vi "RT Driver VI.vi"(6 "Device Clock":string, 9 "Device Inputs FIFO":refnum<k33>, 10 "Device Outputs FIFO":refnum<k33>, 11 "Device Reference":T1 format="%.0x") -> ()   [LabVIEW 2019, in "DeltaPSControl Engine.lvlib"]
uses:
  DeltaPSControl Engine.lvlib
  <vilib>/NI VeriStand/Custom Device API/Custom Device Item Ref.ctl
  <vilib>/NI VeriStand/Custom Device API/Custom Device Channel Type.ctl
  <vilib>/NI VeriStand/Custom Device API/Message Response (String).ctl
  <vilib>/NI VeriStand/Custom Device API/Message Response (Byte Array).ctl
  Shared/Constants.vi
  <vilib>/NI VeriStand/Custom Device API/Get Item Property (String Array).vi
  <vilib>/NI VeriStand/Custom Device API/Get Item Property (String).vi
  <vilib>/NI VeriStand/Custom Device API/Get Item Property (U16).vi
  <vilib>/NI VeriStand/Custom Device API/Custom Device API.lvlib
  <vilib>/NI VeriStand/Custom Device Tools/Custom Device Utility Library/Custom Device Utility Library.lvlib
  Shared/DeltaPSControl Shared.lvlib
panel:
  out "idn/pud":string
  in  "Initialization Status Notifier":refnum<notifier>
  in  "Status Notifier":refnum<notifier>
  # "Custom Device Template\nv1.0"
  # "Use this template as a starting point for creating a custom device code module. The input controls shown here are specially named controls that the system will use to provide the device loop with data. The controls are not required for the device loop to run. For instance, if the device doesn't produce any output data, then you don't need the Device Outputs FIFO control. If you do use these controls, however, they need to have these exact names to be functional."
  # "The optional status notifier element is used to notify the RT engine of the last state of the custom device, and to indicate the device has completed execution. If this control is not used, a default No Error value is returned to the system when the device finishes execution.\n\nNote: This error state is not checked until the system shuts down. Use an output status channel to send more immediate status values to the system."
  # "This optional input can be used to send the VeriStand Engine the final status of the custom device initalization process. If this control exists on the custom device front panel, the VeriStand Engine will wait for a status update before starting up. If the custom device reports an error, that will abort the execution of the current configuration in the VeriStand Engine.\n\nThis control can be deleted if the custom device does not need to send the initialization status update."
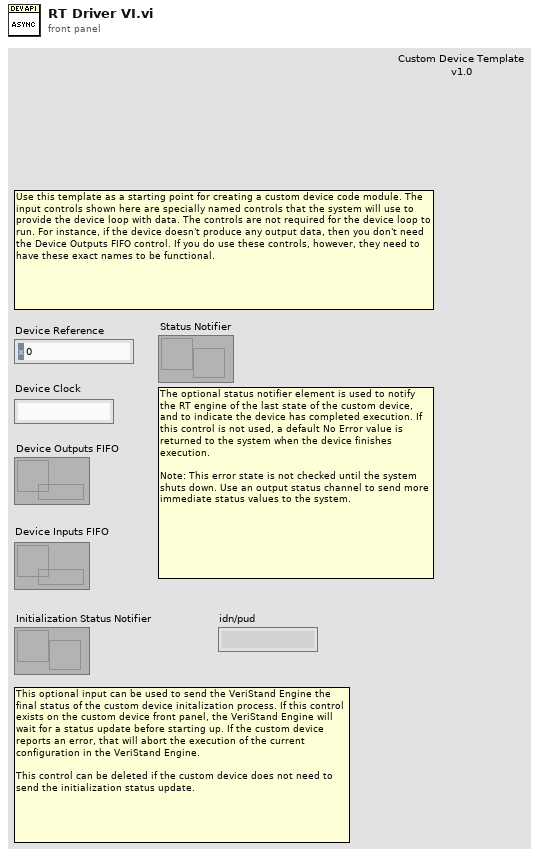
[diagram p1: front panel]
types:
  T1 = typedef "Custom Device API.lvlib/Custom Device Item Ref.ctl" = u64
  T2 = typedef "Custom Device API.lvlib/Custom Device Channel Type.ctl" = enum16{"Input", "Output"}
  T3 = typedef "Custom Device API.lvlib/Custom Device Engine Event Ref.ctl" = refnum<event-registration>
  T4 = cluster{"Input Values":dbl[], "Device Error":errorcluster, "connection ID":refnum<k5>, "First_Time":bool, "Seq List":string[]}
  T5 = typedef "Custom Device API.lvlib/Message Response (String).ctl" = cluster{"Response":string, "Error":errorcluster}
  T6 = typedef "Custom Device API.lvlib/Message Response (Byte Array).ctl" = cluster{"Response":u8[], "Error":errorcluster}
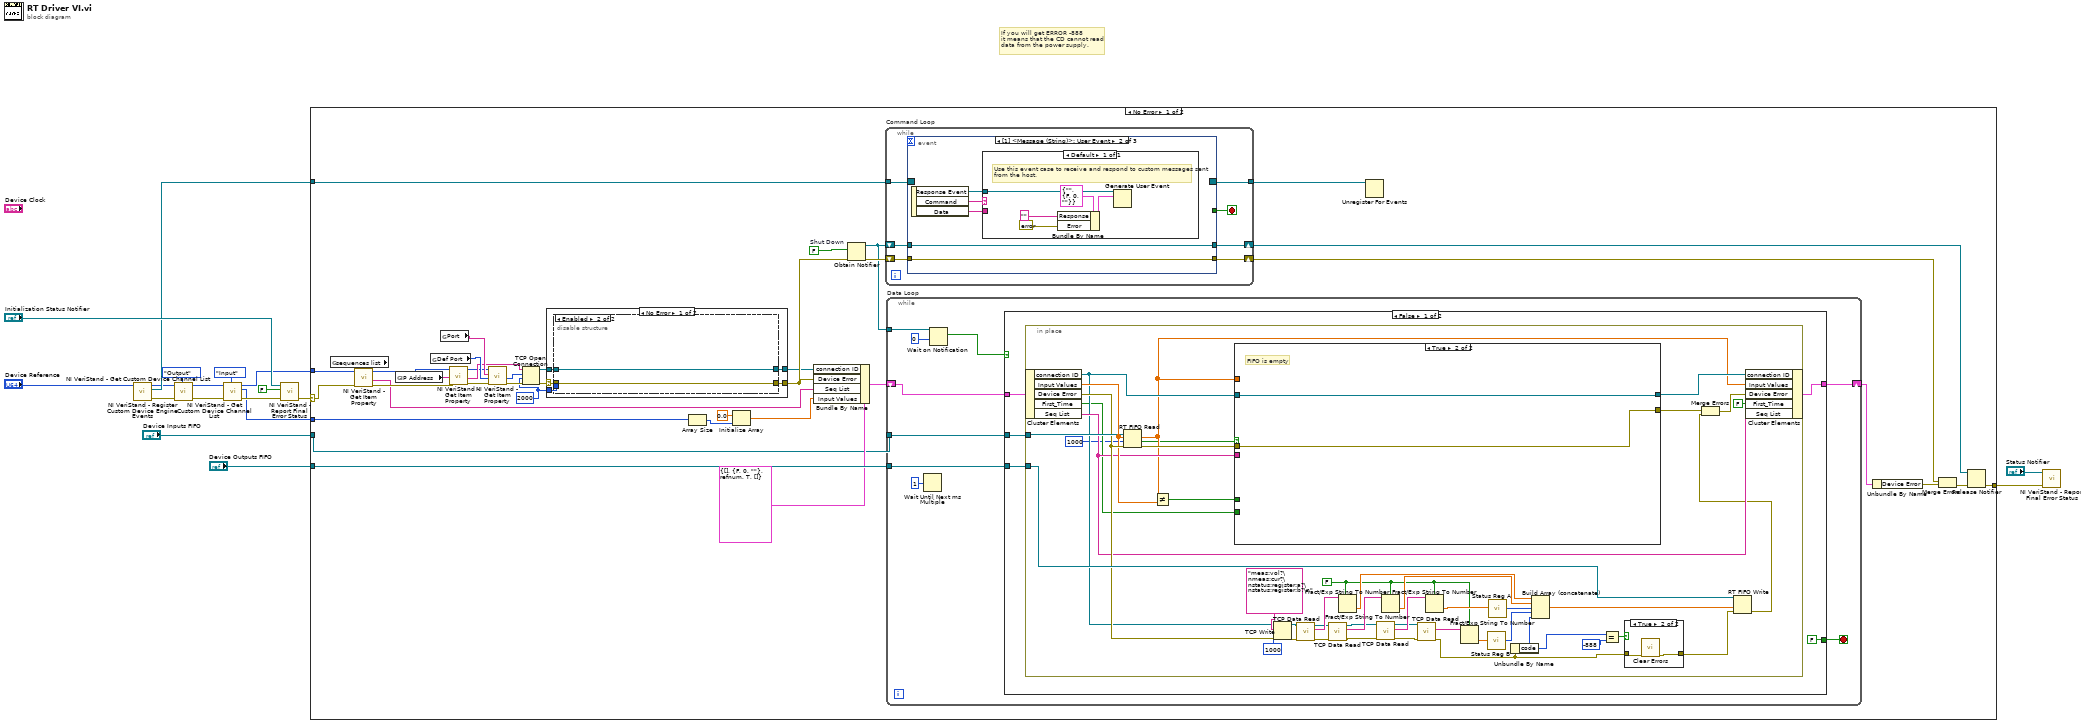
[diagram p0: block diagram]
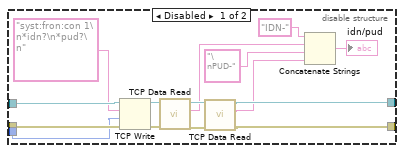
[diagram p2: hidden frame]
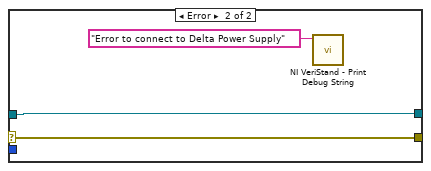
[diagram p3: hidden frame]
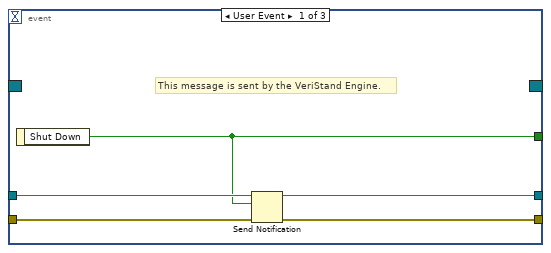
[diagram p4: hidden frame]
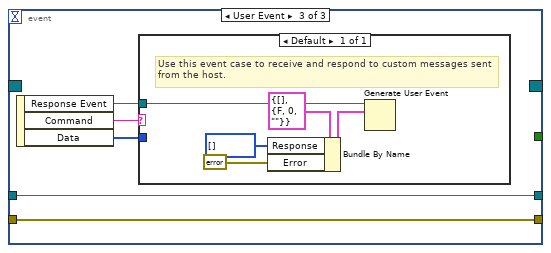
[diagram p5: hidden frame]
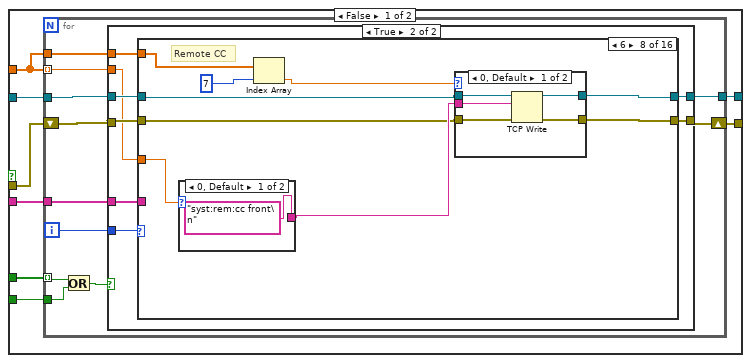
[diagram p6: hidden frame]
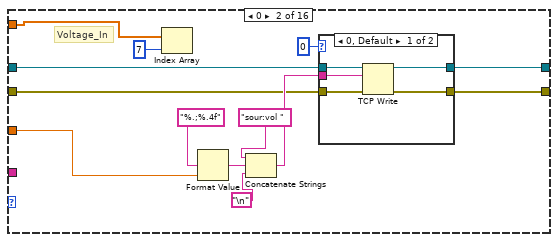
[diagram p9: hidden frame]
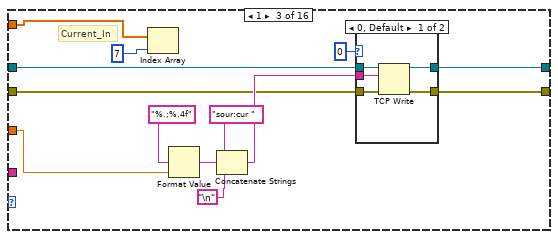
[diagram p11: hidden frame]
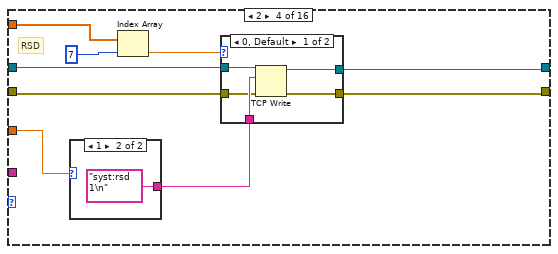
[diagram p13: hidden frame]
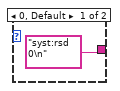
[diagram p15: hidden frame]
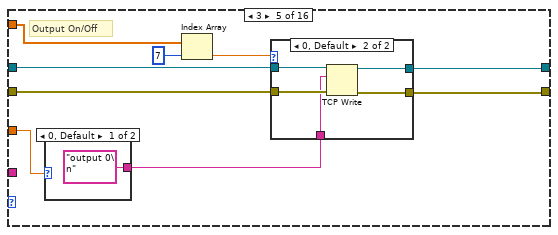
[diagram p16: hidden frame]
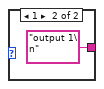
[diagram p18: hidden frame]
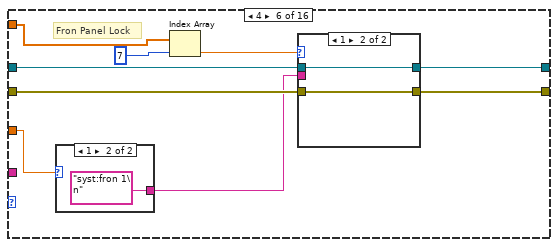
[diagram p19: hidden frame]
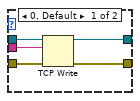
[diagram p20: hidden frame]
diagram:
  # "If you will get ERROR -888\nit means that the CD cannot read \ndata from the power supply."
  n1 = call <vilib>:"NI VeriStand - Register Custom Device Engine Events.vi"("Device Ref in"="Device Reference") -> ("error out"=w18:errorcluster, "Custom Device Engine Event Ref"=w8:T3, "Device Ref out"=w5:T1)  [unwired: 8 in]
  n2 = call <vilib>:"NI VeriStand - Get Custom Device Channel List.vi"("Channel Type"=Custom_Device_Channel_Type."Output", "error in (no error)"=w18, "Device Ref in"=w5) -> ("error out"=w11:errorcluster, "Device Ref out"=w12:T1)  [unwired: 7 out]
  n3 = call <vilib>:"NI VeriStand - Get Custom Device Channel List.vi"("Channel Type"=Custom_Device_Channel_Type."Input", "error in (no error)"=w11, "Device Ref in"=w12) -> ("error out"=w17:errorcluster, "Specified Channel Ref List"=w1:T1[], "Device Ref out"=w2:T1)  [unwired: 6 out]
  n4 = call <vilib>:"NI VeriStand - Report Final Error Status.vi"("error in (no error)"=w17, "Filter FIFO & Shutdown Errors (T)"=FALSE ("Filter FIFO Errors (T)"), "Status Notifier"="Initialization Status Notifier") -> ("error out"=w4:errorcluster)  [unwired: 8 out]
  n5 = case shown="No Error" w4 {
    selector: w4 -> [w28 w494]
    tunnel: "Device Outputs FIFO" -> [w55 _]
    tunnel: "Device Inputs FIFO" -> [w20 _]
    tunnel: w8 -> [w54 _]
    tunnel: [w52 w494] -> w7
    tunnel: w2 -> [w27 _]
    tunnel: w1 -> [w34 _]
    frame No Error {
      w36 = 2000 ("timeout ms (60000)")
      w53 = FALSE  # Shut Down
      n6 = global read "Constants.vi" "sequences list"() -> (w31:string)
      n7 = call-poly <vilib>:"NI VeriStand - Get Item Property.vi"("error in (no error)"=w28, "Property Name"=w31, "Item Ref in"=w27) -> ("error out"=w29:errorcluster, "Value"=w26:string[], "Item Ref out"=w30:T1)  [unwired: 5 in, 1 out]
      n8 = global read "Constants.vi" "IP Address"() -> (w44:string)
      n9 = global read "Constants.vi" "Def Port"() -> (w46:u16)
      n10 = global read "Constants.vi" "Port"() -> (w45:string)
      n11 = call-poly <vilib>:"NI VeriStand - Get Item Property.vi"("error in (no error)"=w29, "Property Name"=w44, "Item Ref in"=w30) -> ("error out"=w38:errorcluster, "Value"=w41:string, "Item Ref out"=w37:T1)  [unwired: 5 in, 1 out]
      n12 = call-poly <vilib>:"NI VeriStand - Get Item Property.vi"("error in (no error)"=w38, "Default Value"=w46, "Property Name"=w45, "Item Ref in"=w37) -> ("error out"=w39:errorcluster, "Value"=w42:u16)  [unwired: 4 in, 2 out]
      n13 = TCP Open Connection(address=w41, remote port or service name=w42, timeout ms (60000)=w36, error in (no error)=w39) -> (connection ID=w40:refnum<k5>, error out=w43:errorcluster)  [unwired: 1 in]
      n14 = case shown="No Error" w43 {
        selector: w43 -> [w60 w81]
        tunnel: w40 -> [w61 w79]
        tunnel: [w58 w79] -> w24
        tunnel: [w57 w81] -> w25
        tunnel: w36 -> [w59 _]
        frame No Error {
          n15 = disable-structure shown="Enabled" {
            disable-tunnel: w61 -> [w76 w78]
            disable-tunnel: w60 -> [w72 w77]
            disable-tunnel: w59 -> [w71 _]
            disable-tunnel: [w66 w78] -> w58
            disable-tunnel: [w65 w77] -> w57
            frame Disabled {
              n16 = TCP Write(connection ID=w76, data in="syst:fron:con 1\n*idn?\n*pud?\n", error in (no error)=w72, 9:w71) -> (connection ID out=w69:refnum<k5>, error out=w68:errorcluster)  [unwired: 1 out]
              n17 = call "TCP Data Read.vi"("error in (no error)"=w68, "Connection ID in"=w69) -> ("error out"=w64:errorcluster, "TCP Read data"=w63:string, "Connection ID out"=w67:refnum<k5>)  [unwired: 6 in, 1 out]
              n18 = call "TCP Data Read.vi"("error in (no error)"=w64, "Connection ID in"=w67) -> ("error out"=w65:errorcluster, "TCP Read data"=w62:string, "Connection ID out"=w66:refnum<k5>)  [unwired: 6 in, 1 out]
              n19 = Concatenate Strings("IDN-" ("string"), w63, "\nPUD-" ("string"), w62) -> (→"idn/pud":string)
            }
            frame Enabled {
            }
          }
        }
        frame Error {
          n20 = call <vilib>:"NI VeriStand - Print Debug String.vi"("Message"="Error to connect to Delta Power Supply") -> ()  [unwired: 10 in, 1 out]
        }
      }
      n21 = Array Size(array=w34) -> (size(s)=w33:i32)
      n22 = Initialize Array(0.0 ("element"), w33) -> (w19:dbl[])
      n23 = Bundle By Name(cluster=T4 {"Input Values"=[], "Device Error"={"status"=FALSE, "code"=0, "source"=""}, "connection ID"=refnum, "First_Time"=TRUE, "Seq List"=[]}, "connection ID"=w24, "Device Error"=w25, "Seq List"=w26, "Input Values"=w19) -> (w23:T4)
      n24 = Obtain Notifier(notification data type=w53, error in (no error)=w25) -> (notifier out=w50:refnum<notifier>, error out=w56:errorcluster)  [unwired: 2 in, 1 out]
      n25 = while "Command Loop" {
        tunnel: w54 -> [w88]
        tunnel: [w87] -> w51
        shift-right: [w84] -> w49
        shift-left: w50 -> [w85]
        shift-right: [w82] -> w47
        shift-left: w56 -> [w83]
        stop <- w86 stop-if-true
        n26 = event shown="[1] <Message (String)>: User Event" {
          selector: w88 -> [_ _ _]
          dyn-events: [_ _ _] -> w87
          timeout: _ -> [_ _ _]
          tunnel: [w91 _ _] -> w86
          tunnel: w85 -> [w92 w96 w106]
          tunnel: [w93 w96 w106] -> w84
          tunnel: w83 -> [w90 w94 w104]
          tunnel: [w89 w94 w104] -> w82
          event User Event {
            # "This message is sent by the VeriStand Engine."
            n27 = event-data() -> ("Shut Down"=w91:bool)  [unwired: 1 in]
            n28 = Send Notification(notification=w91, notifier=w92, error in (no error)=w90) -> (notifier out=w93:refnum<notifier>, error out=w89:errorcluster)
          }
          event User Event {
            n29 = event-data() -> ("Response Event"=w95:refnum<user-event>, "Command"=w98:string, "Data"=w97:string)  [unwired: 1 in]
            n30 = case shown="Default" w98 {
              tunnel: w97 -> [_]
              tunnel: w95 -> [w103]
              frame Default {
                # "Use this event case to receive and respond to custom messages sent from the host."
                n31 = Bundle By Name(cluster=T5 {"Response"="", "Error"={"status"=FALSE, "code"=0, "source"=""}} ("event data"), "Response"="", "Error"=errorcluster {"status"=FALSE, "code"=0, "source"=""}) -> (w101:T5)
                n32 = Generate User Event(user event=w103, event data cluster=w101) -> ()  [unwired: 2 in, 2 out]
              }
            }
          }
          event User Event {
            n33 = event-data() -> ("Response Event"=w105:refnum<user-event>, "Command"=w108:string, "Data"=w107:u8[])  [unwired: 1 in]
            n34 = case shown="Default" w108 {
              tunnel: w107 -> [_]
              tunnel: w105 -> [w113]
              frame Default {
                # "Use this event case to receive and respond to custom messages sent from the host."
                n35 = Bundle By Name(cluster=T6 {"Response"=[], "Error"={"status"=FALSE, "code"=0, "source"=""}} ("event data"), "Response"=u8[] [], "Error"=errorcluster {"status"=FALSE, "code"=0, "source"=""}) -> (w110:T6)
                n36 = Generate User Event(user event=w113, event data cluster=w110) -> ()  [unwired: 2 in, 2 out]
              }
            }
          }
        }
      }
      n37 = while "Data Loop" {
        tunnel: w55 -> [w117]
        tunnel: w20 -> [w116]
        tunnel: w50 -> [w121]
        shift-right: [w119] -> w22
        shift-left: w23 -> [w120]
        stop <- w118 stop-if-true
        n38 = Wait Until Next ms Multiple(millisecond multiple=u32 1) -> ()  [unwired: 1 out]
        n39 = Wait on Notification(notifier=w121, timeout in ms (-1)=0) -> (notification=w114:bool)  [unwired: 2 in, 3 out]
        n40 = case shown="False" w114 {
          tunnel: w120 -> [w126 w471]
          tunnel: [w123 w470] -> w119
          tunnel: [FALSE TRUE] -> w118
          tunnel: w117 -> [w125 w467]
          tunnel: w116 -> [w124 w468]
          frame False {
            n41 = in-place {
              in-place-border: w125 -> [w152]
              in-place-border: w124 -> [w149]
              w131 = FALSE ("use system decimal point (T)")
              n42 = in-place-cluster #1(w126) -> ("connection ID"=w139:refnum<k5>, "Input Values"=w146:dbl[], "Device Error"=w148:errorcluster, "First_Time"=w132:bool, "Seq List"=w145:string[])
              n43 = RT FIFO Read(0:w149, 1:w146, 2:1000 ("timeout in ms (0)"), 3:w148) -> (9:w130:dbl[], 10:w128:bool, 11:w143:errorcluster)  [unwired: 2 out]
              n44 = Not Equal?(x=w130, y=w146) -> (x != y?=w147:bool[])
              n45 = case shown="True" w128 {
                tunnel: w147 -> [w179 _]
                tunnel: w145 -> [w178 _]
                tunnel: w143 -> [w177 w462]
                tunnel: [w176 w463] -> w142
                tunnel: [w175 w462] -> w141
                tunnel: w139 -> [w174 w463]
                tunnel: w132 -> [w173 _]
                tunnel: w130 -> [w172 _]
                frame False {
                  n46 = for {
                    tunnel: w179 -> [w183] mode=indexing
                    tunnel: w174 -> [w189]
                    tunnel: [w188] -> w176
                    shift-right: [w187] -> w175
                    shift-left: w177 -> [w186]
                    tunnel: w172 -> [w185] mode=indexing
                    tunnel: w173 -> [w182]
                    tunnel: w178 -> [w181]
                    tunnel: w172 -> [w180]
                    i -> [w190]
                    n47 = Or(x=w183, y=w182) -> (x .or. y?=w184:bool)
                    n48 = case shown="True" w184 {
                      tunnel: w190 -> [_ w200]
                      tunnel: w189 -> [w191 w199]
                      tunnel: [w191 w198] -> w188
                      tunnel: [w192 w197] -> w187
                      tunnel: w186 -> [w192 w196]
                      tunnel: w185 -> [_ w195]
                      tunnel: w181 -> [_ w194]
                      tunnel: w180 -> [_ w193]
                      frame False {
                        # "No Change"
                      }
                      frame True {
                        n49 = case shown="6" w200 {
                          tunnel: w199 -> [w202 w210 w230 w250 w269 w287 w305 w318 w334 w343 w369 w381 w393 w405 w417 w441]
                          tunnel: [w202 w209 w228 w246 w267 w286 w304 w317 w334 w339 w367 w379 w391 w403 w415 w440] -> w198
                          tunnel: [w201 w208 w227 w247 w266 w284 w303 w316 w333 w338 w366 w378 w390 w402 w414 w439] -> w197
                          tunnel: w196 -> [w201 w207 w229 w248 w268 w285 w302 w319 w333 w342 w368 w380 w392 w404 w416 w438]
                          tunnel: w195 -> [_ w206 w226 w251 w265 w282 w300 w323 _ w336 w365 w377 w389 w401 w413 _]
                          tunnel: w194 -> [_ _ _ _ _ _ _ _ _ w335 _ _ _ _ _ _]
                          tunnel: w193 -> [_ w205 w224 w244 w263 w280 w298 w321 _ _ _ _ _ _ _ w426]
                          frame -1, Default {
                            # "Default"
                          }
                          frame 0 {
                            # "Voltage_In"
                            n50 = Index Array(array=w205, index=7) -> ()  [unwired: 1 out]
                            n51 = Format Value(format string="%.;%.4f", value (0)=w206) -> (output string=w215:string)  [unwired: 1 out]
                            n52 = Concatenate Strings("sour:vol " ("string"), w215, "\n") -> (w211:string)
                            n53 = case shown="0, Default" 0 {
                              tunnel: w211 -> [w220 _]
                              tunnel: w210 -> [w219 w222]
                              tunnel: [w218 w222] -> w209
                              tunnel: [w217 w221] -> w208
                              tunnel: w207 -> [w216 w221]
                              frame 0, Default {
                                n54 = TCP Write(connection ID=w219, data in=w220, error in (no error)=w216) -> (connection ID out=w218:refnum<k5>, error out=w217:errorcluster)  [unwired: 2 out]
                              }
                              frame 1 {
                              }
                            }
                          }
                          frame 1 {
                            # "Current_In"
                            n55 = Index Array(array=w224, index=7) -> ()  [unwired: 1 out]
                            n56 = Format Value(format string="%.;%.4f", value (0)=w226) -> (output string=w235:string)  [unwired: 1 out]
                            n57 = Concatenate Strings("sour:cur " ("string"), w235, "\n") -> (w231:string)
                            n58 = case shown="0, Default" 0 {
                              tunnel: w231 -> [w240 _]
                              tunnel: w230 -> [w239 w242]
                              tunnel: w229 -> [w238 w241]
                              tunnel: [w237 w242] -> w228
                              tunnel: [w236 w241] -> w227
                              frame 0, Default {
                                n59 = TCP Write(connection ID=w239, data in=w240, error in (no error)=w238) -> (connection ID out=w237:refnum<k5>, error out=w236:errorcluster)  [unwired: 2 out]
                              }
                              frame 1 {
                              }
                            }
                          }
                          frame 2 {
                            # "RSD"
                            n60 = case shown="1" w251 {
                              tunnel: ["syst:rsd 0\n" ("string") "syst:rsd 1\n" ("string")] -> w249
                              frame 0, Default {
                              }
                              frame 1 {
                              }
                            }
                            n61 = Index Array(array=w244, index=7) -> (element=w243:dbl)
                            n62 = case shown="0, Default" w243 {
                              tunnel: w250 -> [w256 w258]
                              tunnel: w249 -> [w255 _]
                              tunnel: w248 -> [w254 w257]
                              tunnel: [w253 w257] -> w247
                              tunnel: [w252 w258] -> w246
                              frame 0, Default {
                                n63 = TCP Write(connection ID=w256, data in=w255, error in (no error)=w254) -> (connection ID out=w252:refnum<k5>, error out=w253:errorcluster)  [unwired: 2 out]
                              }
                              frame 1 {
                              }
                            }
                          }
                          frame 3 {
                            # "Output On/Off"
                            n64 = case shown="0, Default" w265 {
                              tunnel: ["output 0\n" ("string") "output 1\n" ("string")] -> w264
                              frame 0, Default {
                              }
                              frame 1 {
                              }
                            }
                            n65 = Index Array(array=w263, index=7) -> (element=w261:dbl)
                            n66 = case shown="0, Default" w261 {
                              tunnel: w269 -> [w271 w276]
                              tunnel: w268 -> [w270 w275]
                              tunnel: [w271 w274] -> w267
                              tunnel: [w270 w273] -> w266
                              tunnel: w264 -> [_ w272]
                              frame 1 {
                              }
                              frame 0, Default {
                                n67 = TCP Write(connection ID=w276, data in=w272, error in (no error)=w275) -> (connection ID out=w274:refnum<k5>, error out=w273:errorcluster)  [unwired: 2 out]
                              }
                            }
                          }
                          frame 4 {
                            # "Fron Panel Lock"
                            n68 = case shown="1" w282 {
                              tunnel: ["syst:fron 0\n" ("string") "syst:fron 1\n" ("string")] -> w283
                              frame 0, Default {
                              }
                              frame 1 {
                              }
                            }
                            n69 = Index Array(array=w280, index=7) -> (element=w279:dbl)
                            n70 = case shown="1" w279 {
                              tunnel: w287 -> [w292 w294]
                              tunnel: [w291 w294] -> w286
                              tunnel: w285 -> [w290 w293]
                              tunnel: [w289 w293] -> w284
                              tunnel: w283 -> [w288 _]
                              frame 0, Default {
                                n71 = TCP Write(connection ID=w292, data in=w288, error in (no error)=w290) -> (connection ID out=w291:refnum<k5>, error out=w289:errorcluster)  [unwired: 2 out]
                              }
                              frame 1 {
                              }
                            }
                          }
                          frame 5 {
                            # "Remote CV"
                            n72 = case shown="0, Default" w300 {
                              tunnel: ["syst:rem:cv front\n" ("string") "syst:rem:cv eth\n" ("string")] -> w301
                              frame 0, Default {
                              }
                              frame 1 {
                              }
                            }
                            n73 = Index Array(array=w298, index=7) -> (element=w297:dbl)
                            n74 = case shown="1" w297 {
                              tunnel: w305 -> [w310 w312]
                              tunnel: [w309 w312] -> w304
                              tunnel: [w308 w311] -> w303
                              tunnel: w302 -> [w307 w311]
                              tunnel: w301 -> [w306 _]
                              frame 0, Default {
                                n75 = TCP Write(connection ID=w310, data in=w306, error in (no error)=w307) -> (connection ID out=w309:refnum<k5>, error out=w308:errorcluster)  [unwired: 2 out]
                              }
                              frame 1 {
                              }
                            }
                          }
                          frame 6 {
                            # "Remote CC"
                            n76 = case shown="0, Default" w323 {
                              tunnel: ["syst:rem:cc front\n" ("string") "syst:rem:cc eth\n" ("string")] -> w320
                              frame 0, Default {
                              }
                              frame 1 {
                              }
                            }
                            n77 = Index Array(array=w321, index=7) -> (element=w315:dbl)
                            n78 = case shown="0, Default" w315 {
                              tunnel: w318 -> [w328 w330]
                              tunnel: [w327 w330] -> w317
                              tunnel: [w326 w329] -> w316
                              tunnel: w319 -> [w325 w329]
                              tunnel: w320 -> [w324 _]
                              frame 0, Default {
                                n79 = TCP Write(connection ID=w328, data in=w324, error in (no error)=w325) -> (connection ID out=w327:refnum<k5>, error out=w326:errorcluster)  [unwired: 2 out]
                              }
                              frame 1 {
                              }
                            }
                          }
                          frame 7 {
                          }
                          frame 8 {
                            n80 = Array Size(array=w335) -> (size(s)=w341:i32)
                            n81 = Greater?(x=w341, y=0) -> (0:w337:bool)
                            n82 = case shown="True" w337 {
                              tunnel: w343 -> [w345 w354]
                              tunnel: w342 -> [w344 w353]
                              tunnel: [w345 w352] -> w339
                              tunnel: [w344 w351] -> w338
                              tunnel: w336 -> [_ w349]
                              tunnel: w335 -> [_ w350]
                              frame False {
                              }
                              frame True {
                                n83 = Index Array(array=w350, index=w349) -> (element=w348:string)
                                n84 = Not Equal?(x=w348, y="") -> (x != y?=w347:bool)
                                n85 = case shown="True" w347 {
                                tunnel: w354 -> [w356 w364]
                                tunnel: w353 -> [w355 w363]
                                tunnel: [w356 w362] -> w352
                                tunnel: [w355 w361] -> w351
                                tunnel: w348 -> [_ w358]
                                frame False {
                                }
                                frame True {
                                n86 = Concatenate Strings("prog:sel:nam " ("data in"), w358, "\n") -> (w357:string)
                                n87 = TCP Write(connection ID=w364, data in=w357, error in (no error)=w363) -> (connection ID out=w362:refnum<k5>, error out=w361:errorcluster)  [unwired: 2 out]
                                }
                                }
                              }
                            }
                          }
                          frame 9 {
                            # "Trigger seq"
                            n88 = case shown="0, Default" w365 {
                              tunnel: w369 -> [w371 w375]
                              tunnel: w368 -> [w370 w374]
                              tunnel: [w371 w373] -> w367
                              tunnel: [w370 w372] -> w366
                              frame 0, Default {
                              }
                              frame 1 {
                                n89 = TCP Write(connection ID=w375, data in="trig:imm\n" ("string"), error in (no error)=w374) -> (connection ID out=w373:refnum<k5>, error out=w372:errorcluster)  [unwired: 2 out]
                              }
                            }
                          }
                          frame 10 {
                            # "Start seq"
                            n90 = case shown="1" w377 {
                              tunnel: w381 -> [w383 w387]
                              tunnel: w380 -> [w382 w386]
                              tunnel: [w383 w385] -> w379
                              tunnel: [w382 w384] -> w378
                              frame 0, Default {
                              }
                              frame 1 {
                                n91 = TCP Write(connection ID=w387, data in="prog:sel:sta run\n" ("string"), error in (no error)=w386) -> (connection ID out=w385:refnum<k5>, error out=w384:errorcluster)  [unwired: 2 out]
                              }
                            }
                          }
                          frame 11 {
                            # "Pause seq"
                            n92 = case shown="0, Default" w389 {
                              tunnel: w393 -> [w395 w399]
                              tunnel: w392 -> [w394 w398]
                              tunnel: [w395 w397] -> w391
                              tunnel: [w394 w396] -> w390
                              frame 0, Default {
                              }
                              frame 1 {
                                n93 = TCP Write(connection ID=w399, data in="prog:sel:sta paus\n" ("string"), error in (no error)=w398) -> (connection ID out=w397:refnum<k5>, error out=w396:errorcluster)  [unwired: 2 out]
                              }
                            }
                          }
                          frame 12 {
                            # "Continue seq"
                            n94 = case shown="0, Default" w401 {
                              tunnel: w405 -> [w407 w411]
                              tunnel: w404 -> [w406 w410]
                              tunnel: [w407 w409] -> w403
                              tunnel: [w406 w408] -> w402
                              frame 0, Default {
                              }
                              frame 1 {
                                n95 = TCP Write(connection ID=w411, data in="prog:sel:sta cont\n" ("string"), error in (no error)=w410) -> (connection ID out=w409:refnum<k5>, error out=w408:errorcluster)  [unwired: 2 out]
                              }
                            }
                          }
                          frame 13 {
                            # "Stop seq"
                            n96 = case shown="0, Default" w413 {
                              tunnel: w417 -> [w419 w423]
                              tunnel: w416 -> [w418 w422]
                              tunnel: [w419 w421] -> w415
                              tunnel: [w418 w420] -> w414
                              frame 0, Default {
                              }
                              frame 1 {
                                n97 = TCP Write(connection ID=w423, data in="prog:sel:sta stop\n" ("string"), error in (no error)=w422) -> (connection ID out=w421:refnum<k5>, error out=w420:errorcluster)  [unwired: 2 out]
                              }
                            }
                          }
                          frame 14, 15 {
                            w433 = ""
                            w436 = "front\nweb\nsequencer\nethernet" ("multi-line string")
                            # "Current mode"
                            # "Voltage mode"
                            n98 = Index Array(array=w426, index=7) -> (element=w425:dbl)
                            n99 = Index Array(array=w426, index #1=14 ("index")) -> (element #1=w435:dbl, element #2=w434:dbl)  [unwired: 1 in]
                            n100 = Pick Line(multi-line string=w436, line index=w435) -> (output string=w429:string)  [unwired: 1 in]
                            n101 = Pick Line(multi-line string=w436, line index=w434) -> (output string=w428:string)  [unwired: 1 in]
                            n102 = Not Equal?(x=w429, y=w433) -> (x != y?=w432:bool)
                            n103 = Not Equal?(x=w433, y=w428) -> (x != y?=w431:bool)
                            n104 = And(x=w432, y=w431) -> (x .and. y?=w430:bool)
                            n105 = case shown="True" w430 {
                              tunnel: w441 -> [w442 w447]
                              tunnel: [w442 w453] -> w440
                              tunnel: [w443 w452] -> w439
                              tunnel: w438 -> [w443 w451]
                              tunnel: w429 -> [_ w450]
                              tunnel: w428 -> [_ w448]
                              tunnel: w425 -> [_ w444]
                              frame False {
                              }
                              frame True {
                                n106 = Concatenate Strings("prog:sou " ("string"), w450, "," ("string"), w448, "\n") -> (w445:string)
                                n107 = case shown="0, Default" w444 {
                                tunnel: [w459 w461] -> w453
                                tunnel: [w458 w460] -> w452
                                tunnel: w451 -> [w457 w460]
                                tunnel: w447 -> [w456 w461]
                                tunnel: w445 -> [w455 _]
                                frame 0, Default {
                                n108 = TCP Write(connection ID=w456, data in=w455, error in (no error)=w457) -> (connection ID out=w459:refnum<k5>, error out=w458:errorcluster)  [unwired: 2 out]
                                }
                                frame 1 {
                                }
                                }
                              }
                            }
                          }
                        }
                      }
                    }
                  }
                }
                frame True {
                  # "FIFO is empty"
                }
              }
              n109 = TCP Write(connection ID=w139, data in="meas:vol?\nmeas:cur?\nstatus:register:a?\nstatus:register:b?\n", error in (no error)=w148, 9:1000) -> (connection ID out=w169:refnum<k5>, error out=w168:errorcluster)  [unwired: 1 out]
              n110 = call "TCP Data Read.vi"("error in (no error)"=w168, "Connection ID in"=w169) -> ("error out"=w165:errorcluster, "TCP Read data"=w167:string, "Connection ID out"=w166:refnum<k5>)  [unwired: 6 in, 1 out]
              n111 = call "TCP Data Read.vi"("error in (no error)"=w165, "Connection ID in"=w166) -> ("error out"=w162:errorcluster, "TCP Read data"=w164:string, "Connection ID out"=w163:refnum<k5>)  [unwired: 6 in, 1 out]
              n112 = Fract/Exp String To Number(use system decimal point (T)=w131, string=w167) -> (number=w171:dbl)  [unwired: 2 in, 1 out]
              n113 = call "TCP Data Read.vi"("error in (no error)"=w162, "Connection ID in"=w163) -> ("error out"=w159:errorcluster, "TCP Read data"=w161:string, "Connection ID out"=w160:refnum<k5>)  [unwired: 6 in, 1 out]
              n114 = Fract/Exp String To Number(use system decimal point (T)=w131, string=w164) -> (number=w170:dbl)  [unwired: 2 in, 1 out]
              n115 = call "TCP Data Read.vi"("error in (no error)"=w159, "Connection ID in"=w160) -> ("error out"=w133:errorcluster, "TCP Read data"=w158:string)  [unwired: 6 in, 2 out]
              n116 = Fract/Exp String To Number(use system decimal point (T)=w131, string=w161) -> (number=w157:dbl)  [unwired: 2 in, 1 out]
              n117 = Fract/Exp String To Number(use system decimal point (T)=w131, string=w158) -> (number=w155:dbl)  [unwired: 2 in, 1 out]
              n118 = call "Status Reg B.vi"("Status:Register:B"=w155) -> ("Reg B"=w154:i16[])
              n119 = call "Status Reg A.vi"("Status:Register:A"=w157) -> ("Reg A"=w156:i16[])
              n120 = Unbundle By Name(w133) -> ("code"=w137:i32)
              n121 = Build Array (concatenate)(w171, w170, w156, w154, w137) -> (w151:dbl[])
              n122 = Equal?(x=w137, y=-888) -> (x = y?=w135:bool)
              n123 = case shown="True" w135 {
                tunnel: w133 -> [w464 w466]
                tunnel: [w464 w465] -> w134
                frame False {
                }
                frame True {
                  n124 = call <vilib>:"Clear Errors.vi"("error in (no error)"=w466) -> ("error out"=w465:errorcluster)  [unwired: 5 in, 1 out]
                }
              }
              n125 = RT FIFO Write(0:w152, 1:w151, 3:w134) -> (11:w138:errorcluster)  [unwired: 1 in, 4 out]
              n126 = Merge Errors(w141, w138) -> (w140:errorcluster)
              n127 = in-place-cluster #1("connection ID"=w142, "Input Values"=w130, "Device Error"=w140, "First_Time"=FALSE, "Seq List"=w145) -> (w123:T4)
            }
          }
          frame True {
            n128 = in-place {
              in-place-border: w468 -> [w476]
              in-place-border: w467 -> [w475]
              n129 = in-place-cluster #2(w471) -> ("connection ID"=w479:refnum<k5>, "Device Error"=w472:errorcluster)
              n130 = disable-structure shown="Disabled" {
                disable-tunnel: w479 -> [w486 w493]
                disable-tunnel: _ -> [w485 _]
                disable-tunnel: [w484 _] -> _
                disable-tunnel: [w483 w493] -> w478
                disable-tunnel: string[] ["syst:rem:cv front\n", "syst:rem:cc front\n", "output 0\n", "syst:fron 0\n", "syst:rsd 0\n"] -> [w482 _]
                frame Disabled {
                  n131 = for {
                    tunnel: w486 -> [w492]
                    shift-right: [w491] -> w484
                    shift-left: w485 -> [w490]
                    tunnel: [w489] -> w483
                    tunnel: w482 -> [w488] mode=indexing
                    n132 = TCP Write(connection ID=w492, data in=w488, error in (no error)=w490, 9:1000 ("timeout ms (25000)")) -> (connection ID out=w489:refnum<k5>, error out=w491:errorcluster)  [unwired: 1 out]
                  }
                }
                frame Enabled {
                }
              }
              n133 = RT FIFO Delete(0:w476, 3:w472) -> (11:w474:errorcluster)  [unwired: 1 in]
              n134 = RT FIFO Delete(0:w475, 3:w474) -> (11:w473:errorcluster)  [unwired: 1 in]
              n135 = TCP Close Connection(connection ID=w478, error in (no error)=w473) -> (connection ID out=w480:refnum<k5>, error out=w481:errorcluster)  [unwired: 1 in]
              n136 = in-place-cluster #2("connection ID"=w480, "Device Error"=w481) -> (w470:T4)
            }
          }
        }
      }
      n137 = Unregister For Events(event registration refnum=w51) -> ()  [unwired: 1 in, 1 out]
      n138 = Unbundle By Name(w22) -> ("Device Error"=w21:errorcluster)
      n139 = Merge Errors(w47, w21) -> (w48:errorcluster)
      n140 = Release Notifier(notifier=w49, error in (no error)=w48) -> (error out=w52:errorcluster)  [unwired: 1 in, 2 out]
    }
    frame Error {
    }
  }
  n141 = call <vilib>:"NI VeriStand - Report Final Error Status.vi"("error in (no error)"=w7, "Status Notifier"="Status Notifier") -> ()  [unwired: 1 in, 9 out]
